vi "automated_scan_v1.2.vi"() -> ()   [LabVIEW 2018]
uses:
  Other_Libraries/MoCo Software/VI/global_m.vi
  <vilib>/Utility/file.llb/Write Delimited Spreadsheet (DBL).vi
  <vilib>/Utility/file.llb/Write Delimited Spreadsheet (string).vi
  Other_Libraries/Thorlabs_FW102C/Thorlabs_FW102C.lvlib
panel:
  out "Time per step":dbl
  out "Scan time(min)":dbl
  out "End scan":errorcluster
  out "FW Position":i32
  out "Filter Wheel":errorcluster
  out "Current Wavelength(nm)":dbl
  out "Take Image":errorcluster
  out "% complete":dbl
  out "Total Steps":dbl
  in  "Tab Control":T1(tab)
  in  "Mono port":refnum<visa-resource-name>="COM2"
  in  "Grating, gr/mm":u16(ring)=2 items=["2400", "1800", "1200", "600", "300", "150"]
  in  "Take Image":bool=TRUE
  in  "Two Cameras":bool=TRUE
  in  "Step Size":dbl=10.0
  in  "Stop Wavelength":dbl=600.0
  in  "Start Wavelength":dbl=500.0
  in  "Scan Directory":string="Peter_ferguson\\Tcal\\scans\\"
  in  "Scan Name":string="test_scan"
  in  "Scan Type":string(combo)="New Scan"
  in  "Camera\n Integration time":dbl=10.0
  in  "Spectrometer Integration time":dbl=0.001
  out "VISA out":refnum<visa-resource-name>
  out "Mono wav":dbl format="%.3f"
  out "Mono/Photodiode":errorcluster
  out "Step #":i32
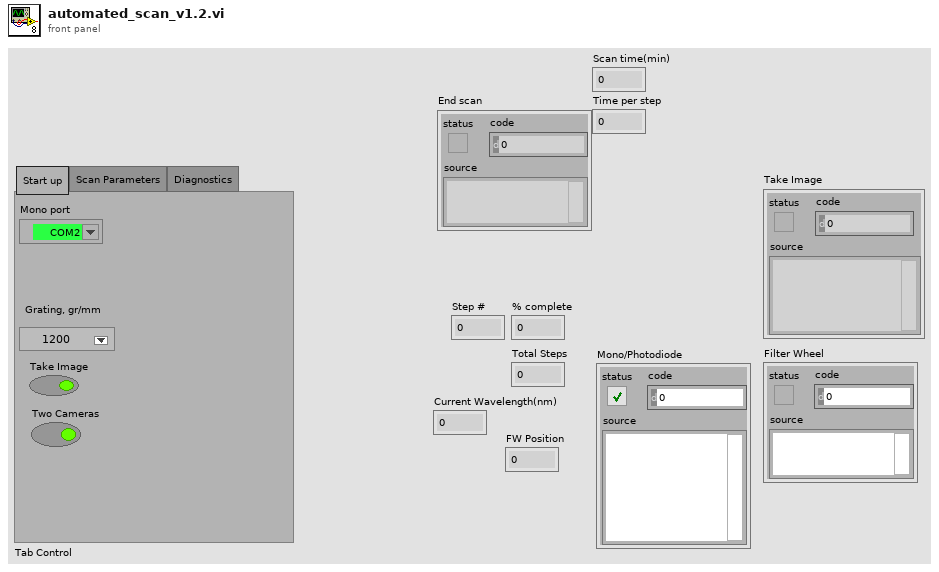
[diagram p1: front panel]
types:
  T1 = enum32{"Start up", "Scan Parameters", "Diagnostics"}
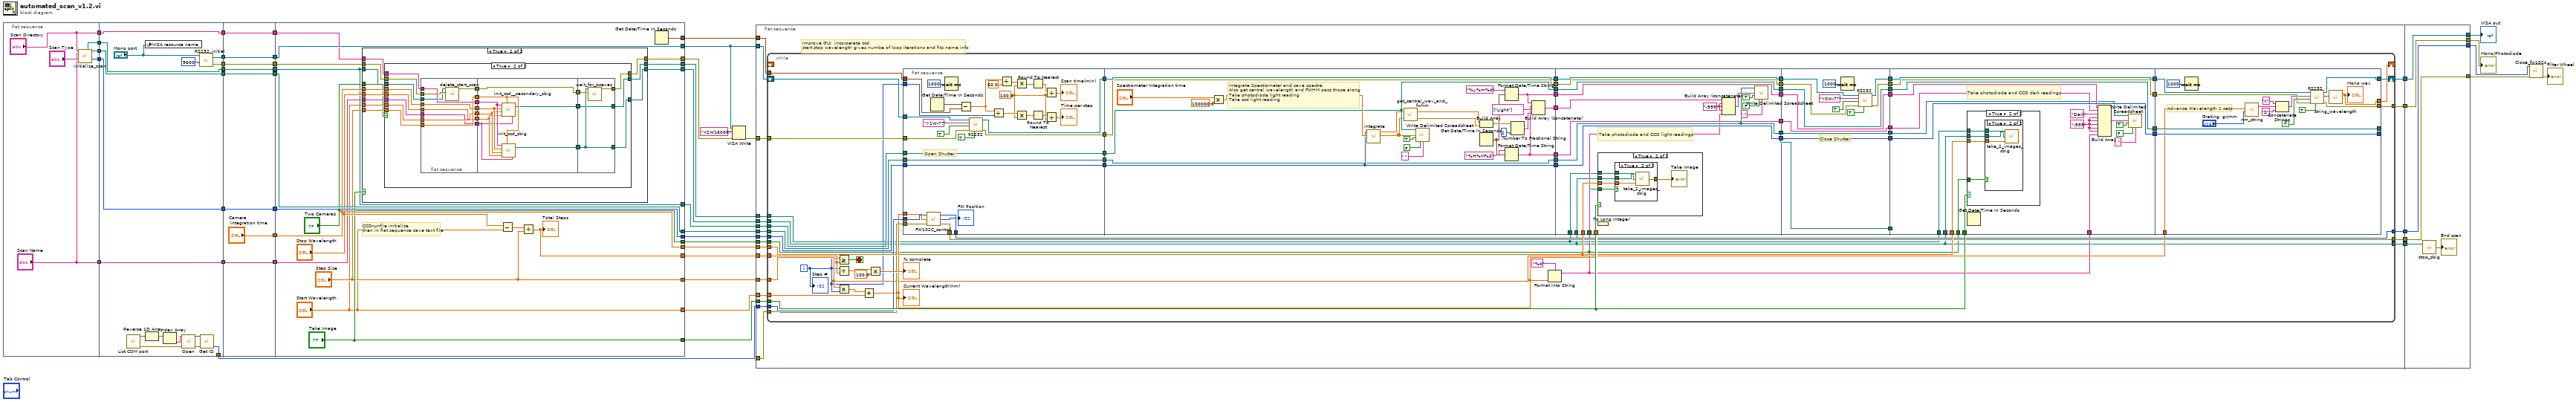
[diagram p0: block diagram]
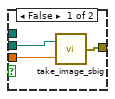
[diagram p3: hidden frame]
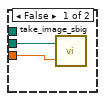
[diagram p5: hidden frame]
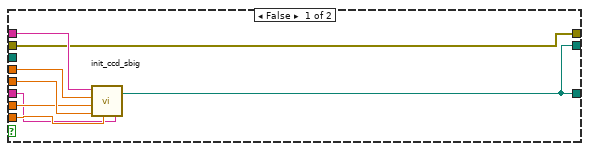
[diagram p7: hidden frame]
diagram:
  n1 = flat-sequence {
    tunnel: [w53] -> w39
    tunnel: [w52] -> w38
    tunnel: [w51] -> w37
    tunnel: ["Scan Directory"] -> w24
    tunnel: ["Scan Name"] -> w10
    tunnel: [w69] -> w36
    tunnel: [w68] -> w35
    tunnel: w39 -> [w67]
    tunnel: [w67] -> w34
    tunnel: w38 -> [w66]
    tunnel: [w66] -> w33
    tunnel: w37 -> [w65]
    tunnel: [w65] -> w32
    tunnel: w24 -> [w64]
    tunnel: [w64] -> w22
    tunnel: [w57] -> w17
    tunnel: [w56] -> w16
    tunnel: [w55] -> w11
    tunnel: w10 -> [w55]
    tunnel: w36 -> [w78]
    tunnel: [w78] -> w31
    tunnel: w35 -> [w72]
    tunnel: w34 -> [w77]
    tunnel: [w77] -> w30
    tunnel: w33 -> [w76]
    tunnel: [w76] -> w29
    tunnel: w32 -> [w75]
    tunnel: [w75] -> w28
    tunnel: ["Camera\n Integration time"] -> w27
    tunnel: [w72] -> w26
    tunnel: [w74] -> w23
    tunnel: w22 -> [w74]
    tunnel: [w73] -> w12
    tunnel: w11 -> [w73]
    tunnel: [w96] -> w41
    tunnel: w31 -> [w96]
    tunnel: [w88] -> w46
    tunnel: w30 -> [w88]
    tunnel: [w95] -> w45
    tunnel: w29 -> [w95]
    tunnel: [w94] -> w44
    tunnel: w28 -> [w94]
    tunnel: [w92] -> w43
    tunnel: w27 -> [w92]
    tunnel: [w97] -> w40
    tunnel: w26 -> [w84]
    tunnel: [w83] -> w25
    tunnel: w23 -> [w93]
    tunnel: [w90] -> w21
    tunnel: ["Take Image"] -> w20
    tunnel: ["Step Size"] -> w19
    tunnel: ["Start Wavelength"] -> w18
    tunnel: w12 -> [w85]
    tunnel: [w82] -> w4
    tunnel: ["Two Cameras"] -> w3
    tunnel: [w80] -> w1
    frame #0 {
      n2 = call "initialize_scan.vi"("Scan Directory"="Scan Directory", "Scan Name"="Scan Name", "Scan Type"="Scan Type") -> ("Path Spec"=w53:path, "Path Scan"=w51:path, "Wrapper Out"=w52:u64)  [unwired: 8 in, 2 out]
    }
    frame #1 {
      n3 = call "List COM port.vi"() -> ("error out"=w58:errorcluster, "COM Ports"=w61:string[])  [unwired: 10 in]
      n4 = global write "global_m.vi" "VISA resource name"("Mono port") -> ()
      n5 = Reverse 1D Array(array=w61) -> (reversed array=w60:string[])
      n6 = Index Array(array=w60) -> (element=w59:string)  [unwired: 1 in]
      n7 = call "Open.vi"("error in (no error)"=w58, "Serial Port"=w59) -> ("error out"=w62:errorcluster, "FW102C out"=w63:i32)  [unwired: 7 in, 1 out]
      n8 = call "RS232_initial.vi"("baud rate"=u32 9600, "VISA resource name"="Mono port") -> ("error out"=w68:errorcluster, "VISA name out"=w69:refnum<visa-resource-name>)  [unwired: 2 in]
      n9 = call "Get ID.vi"("error in (no error)"=w62, "FW102C in"=w63) -> ("error out"=w56:errorcluster, "FW102C out"=w57:i32)  [unwired: 7 in, 1 out]
    }
    frame #2 {
    }
    frame #3 {
      # "CCDrunfile initialize\nthen in flat sequence save text file"
      n10 = case shown="True" "Take Image" {
        tunnel: w93 -> [_ w112]
        tunnel: w92 -> [_ w111]
        tunnel: "Step Size" -> [_ w110]
        tunnel: "Stop Wavelength" -> [_ w109]
        tunnel: [w99 w108] -> w90
        tunnel: "Start Wavelength" -> [_ w107]
        tunnel: w88 -> [w99 w102]
        tunnel: "Two Cameras" -> [_ w106]
        tunnel: w85 -> [_ w105]
        tunnel: w84 -> [w100 w104]
        tunnel: [w100 w103] -> w83
        tunnel: [w99 w101] -> w82
        frame False {
        }
        frame True {
          n11 = case shown="True" w106 {
            tunnel: w112 -> [w120 w139]
            tunnel: w111 -> [w119 w138]
            tunnel: w110 -> [w118 w140]
            tunnel: w109 -> [w117 w136]
            tunnel: [w113 w141] -> w108
            tunnel: w107 -> [w116 w137]
            tunnel: w105 -> [w115 w135]
            tunnel: w104 -> [w114 w126]
            tunnel: [w114 w133] -> w103
            tunnel: w102 -> [_ w123]
            tunnel: [w113 w121] -> w101
            frame False {
              n12 = call "init_ccd_sbig.vi"("Scan Directory"=w120, "Exposure Time"=w119, "Min nm"=w116, "Max nm"=w117, "Step size"=w118, "Scan_prefix"=w115) -> ("Working Directory"=w113:path)
            }
            frame True {
              n13 = flat-sequence {
                tunnel: w135 -> [w145]
                tunnel: w136 -> [w146]
                tunnel: w137 -> [w147]
                tunnel: w138 -> [w148]
                tunnel: w139 -> [w149]
                tunnel: w140 -> [w150]
                tunnel: [w150] -> w132
                tunnel: [w149] -> w131
                tunnel: [w148] -> w130
                tunnel: [w147] -> w129
                tunnel: [w146] -> w128
                tunnel: [w145] -> w127
                tunnel: w126 -> [w144]
                tunnel: [w143] -> w124
                tunnel: w123 -> [w142]
                tunnel: [w153] -> w134
                tunnel: w132 -> [w159]
                tunnel: w131 -> [w158]
                tunnel: w130 -> [w157]
                tunnel: w129 -> [w156]
                tunnel: w128 -> [w155]
                tunnel: w127 -> [w154]
                tunnel: [w152] -> w125
                tunnel: w124 -> [w152]
                tunnel: [w151] -> w122
                tunnel: [w162] -> w141
                tunnel: w134 -> [w162]
                tunnel: [w163] -> w133
                tunnel: w125 -> [w161]
                tunnel: w122 -> [w160]
                tunnel: [w160] -> w121
                frame #0 {
                  n14 = call "delete_start_scan.vi"("error out"=w144, "base path"=w142) -> ("error out 2"=w143:errorcluster)  [unwired: 9 in]
                }
                frame #1 {
                  n15 = call "init_ccd__secondary_sbig.vi"("Scan Directory"=w158, "Exposure Time"=w157, "Min nm"=w156, "Max nm"=w155, "Step size"=w159, "Scan_prefix"=w154) -> ("Working Directory"=w151:path)
                  n16 = call "init_ccd_sbig.vi"("Scan Directory"=w158, "Exposure Time"=w157, "Min nm"=w156, "Max nm"=w155, "Step size"=w159, "Scan_prefix"=w154) -> ("Working Directory"=w153:path)
                }
                frame #2 {
                  n17 = call "wait_for_psexec.vi"("error out"=w161, "base path"=w162) -> ("error out 2"=w163:errorcluster)  [unwired: 9 in]
                }
              }
            }
          }
        }
      }
      n18 = Subtract(x="Stop Wavelength", y="Start Wavelength") -> (x-y=w98:dbl)
      n19 = Divide(x=w98, y="Step Size") -> (x/y=w97:dbl)
      "Total Steps" <- w97
      n20 = Get Date/Time In Seconds() -> (seconds since 1Jan1904=w80:timestamp)
    }
  }
  n21 = VISA Write(VISA resource name=w41, write buffer="X2W1600R", error in (no error)=w25) -> (error out=w47:errorcluster)  [unwired: 2 out]
  n22 = flat-sequence {
    tunnel: w47 -> [w184]
    tunnel: w46 -> [w183]
    tunnel: w45 -> [w182]
    tunnel: w44 -> [w181]
    tunnel: w43 -> [w180]
    tunnel: w41 -> [w177]
    tunnel: w40 -> [w176]
    tunnel: w21 -> [w175]
    tunnel: w20 -> [w174]
    tunnel: w19 -> [w173]
    tunnel: w18 -> [w172]
    tunnel: w17 -> [w171]
    tunnel: w16 -> [w170]
    tunnel: [w179] -> w9
    tunnel: [w178] -> w8
    tunnel: [w169] -> w7
    tunnel: [w168] -> w6
    tunnel: [w167] -> w5
    tunnel: w4 -> [w166]
    tunnel: w3 -> [w165]
    tunnel: w1 -> [w164]
    tunnel: [w395] -> w13
    tunnel: [w396] -> w14
    tunnel: [w397] -> w42
    tunnel: [w398] -> w2
    tunnel: w9 -> [w398]
    tunnel: w8 -> [w397]
    tunnel: w7 -> [w396]
    tunnel: w6 -> [w395]
    tunnel: w5 -> [w394]
    frame #0 {
      # "Improve GUI, incorperate ccd,\nstart stop wavelength gives numbe of loop iterations and fits name info"
      n23 = while {
        tunnel: w184 -> [w246]
        tunnel: [w245] -> w179
        tunnel: w183 -> [w244]
        tunnel: w182 -> [w243]
        shift-right: [w206] -> _
        shift-left: _ -> [_]
        tunnel: w181 -> [w230]
        tunnel: w180 -> [w198]
        shift-right: [w208] -> w178
        shift-left: w177 -> [w207]
        tunnel: w176 -> [w205]
        tunnel: w175 -> [w189]
        tunnel: w174 -> [w201]
        tunnel: w173 -> [w190]
        tunnel: w172 -> [w200]
        tunnel: w171 -> [w196]
        tunnel: w170 -> [w195]
        tunnel: [w193] -> w168
        tunnel: [w192] -> w169
        tunnel: [w189] -> w167
        tunnel: w166 -> [w188]
        tunnel: w165 -> [w187]
        tunnel: w164 -> [w186]
        i -> [w185]
        stop <- w216 stop-if-true
        n24 = Greater Or Equal?(x=w185, y=w205) -> (x >= y?=w216:bool)
        n25 = Divide(x=w185, y=w205) -> (x/y=w204:dbl)
        n26 = Multiply(x=w190, y=w185) -> (x*y=w199:dbl)
        n27 = Add(x=w199, y=w200) -> (x+y=w194:dbl)
        "Current Wavelength(nm)" <- w194
        n28 = Multiply(x=w204, y=100.0) -> (x*y=→"% complete":dbl)
        n29 = flat-sequence {
          tunnel: w246 -> [w276]
          tunnel: [w275] -> w242
          tunnel: [w274] -> w241
          tunnel: [w270] -> w240
          tunnel: w244 -> [w270]
          tunnel: w243 -> [w269]
          tunnel: [w269] -> w239
          tunnel: w230 -> [w268]
          tunnel: [w268] -> w229
          tunnel: w207 -> [w267]
          tunnel: w196 -> [w266]
          tunnel: w195 -> [w265]
          tunnel: w194 -> [w264]
          tunnel: [w263] -> w193
          tunnel: [w262] -> w192
          tunnel: w186 -> [w259]
          tunnel: w185 -> [w258]
          tunnel: w242 -> [w302]
          tunnel: [w302] -> w228
          tunnel: w241 -> [w301]
          tunnel: [w301] -> w227
          tunnel: w240 -> [w293]
          tunnel: [w293] -> w226
          tunnel: w239 -> [w294]
          tunnel: [w294] -> w224
          tunnel: w229 -> [w282]
          tunnel: [w282] -> w222
          tunnel: [w281] -> w221
          tunnel: [w279] -> w215
          tunnel: [w278] -> w210
          tunnel: w228 -> [w320]
          tunnel: w227 -> [w314]
          tunnel: w226 -> [w322]
          tunnel: [w322] -> w225
          tunnel: w224 -> [w321]
          tunnel: [w321] -> w223
          tunnel: w222 -> [w313]
          tunnel: w221 -> [w316]
          tunnel: [w320] -> w220
          tunnel: w198 -> [w309]
          tunnel: [w314] -> w219
          tunnel: [w313] -> w218
          tunnel: w215 -> [w312]
          tunnel: [w312] -> w214
          tunnel: [w311] -> w211
          tunnel: w210 -> [w311]
          tunnel: w189 -> [w310]
          tunnel: w201 -> [w308]
          tunnel: w191 -> [w306]
          tunnel: w194 -> [w307]
          tunnel: w188 -> [w305]
          tunnel: w187 -> [w304]
          tunnel: [w346] -> w238
          tunnel: [w345] -> w236
          tunnel: w225 -> [w341]
          tunnel: [w341] -> w234
          tunnel: [w340] -> w232
          tunnel: w223 -> [w340]
          tunnel: w220 -> [w339]
          tunnel: w219 -> [w338]
          tunnel: w218 -> [w335]
          tunnel: [w335] -> w217
          tunnel: w214 -> [w337]
          tunnel: [w337] -> w213
          tunnel: [w336] -> w212
          tunnel: w211 -> [w336]
          tunnel: [w335] -> w209
          tunnel: w238 -> [w366]
          tunnel: [w366] -> w237
          tunnel: w236 -> [w365]
          tunnel: [w365] -> w235
          tunnel: w234 -> [w364]
          tunnel: [w364] -> w233
          tunnel: w232 -> [w363]
          tunnel: [w363] -> w231
          tunnel: w217 -> [_]
          tunnel: w198 -> [w354]
          tunnel: w213 -> [w357]
          tunnel: w212 -> [w356]
          tunnel: w209 -> [w355]
          tunnel: w189 -> [w353]
          tunnel: w201 -> [w352]
          tunnel: w191 -> [w351]
          tunnel: w188 -> [w350]
          tunnel: w187 -> [w349]
          tunnel: w237 -> [w389]
          tunnel: w235 -> [w390]
          tunnel: w233 -> [w379]
          tunnel: w231 -> [w381]
          tunnel: [w388] -> w208
          tunnel: [w387] -> w245
          tunnel: [w381] -> _
          tunnel: [w379] -> _
          tunnel: [w378] -> w206
          tunnel: w190 -> [w377]
          frame #0 {
            w249 = 100.0 ("y")
            # "Open Shutter"
            n30 = call "FW102C_control.vi"("error in (no error)"=w265, "Current Wavelength"=w264, "FW102C in"=w266) -> ("error out"=w262:errorcluster, "Position"=→"FW Position":i32, "FW102C out"=w263:i32)
            n31 = Get Date/Time In Seconds() -> (seconds since 1Jan1904=w260:timestamp)
            n32 = Wait (ms)(milliseconds to wait=u32 1000) -> ()  [unwired: 1 out]
            n33 = Subtract(x=w260, y=w259) -> (x-y=w257:dbl)
            n34 = call "RS232.vi"("read"=TRUE, "error in"=w276, "write"=TRUE, "string to write"="Y1W-7?" ("string"), "VISA  name in"=w267) -> ("error out"=w274:errorcluster, "VISA out"=w275:refnum<visa-resource-name>)  [unwired: 1 in, 2 out]
            n35 = Divide(x=w257, y=w258) -> (x/y=w255:dbl)
            n36 = Divide(x=w257, y=60.0) -> (x/y=w251:dbl)
            n37 = Multiply(x=w251, y=w249) -> (x*y=w250:dbl)
            n38 = Multiply(x=w255, y=w249) -> (x*y=w254:dbl)
            n39 = Round To Nearest(number=w250) -> (nearest integer value=w248:dbl)
            n40 = Round To Nearest(number=w254) -> (nearest integer value=w253:dbl)
            n41 = Divide(x=w248, y=w249) -> (x/y=→"Scan time(min)":dbl)
            n42 = Divide(x=w253, y=w249) -> (x/y=→"Time per step":dbl)
          }
          frame #1 {
            # "Integrate Spectrometer and save spectra, \nAlso get central wavelength and FWHM pass those along\nTake photodiode light reading \nTake ccd light reading"
            n43 = Multiply(x="Spectrometer Integration time", y=100000.0) -> (x*y=w298:dbl)
            n44 = call "integrate.vi"("Numeric"=w298, "Wrapper Out"=w294) -> ("Spectrum Values"=w291:dbl[], "WL Values"=w292:dbl[])  [unwired: 7 in, 1 out]
            n45 = call "get_central_wav_and_fwhm.vi"("Signal"=w291, "Wavelenghs"=w292) -> ("FWHM"=w287:dbl, "Central"=w280:dbl)
            n46 = call-poly <vilib>:"Write Delimited Spreadsheet.vi"("file path (dialog if empty)"=w293, "1D data"=w291, "append to file? (new file:F)"=TRUE, "transpose? (no:F)"=FALSE, "delimiter (\\t)"="," ("delimiter (\\t)")) -> ()  [unwired: 9 in, 2 out]
            n47 = Build Array(w280, w287) -> (w286:dbl[])
            n48 = Get Date/Time In Seconds() -> (seconds since 1Jan1904=w289:timestamp)
            n49 = Format Date/Time String(time format string (%c)="%y%m%d", seconds (now)=w289) -> (date/time string=w279:string)  [unwired: 1 in]
            n50 = Format Date/Time String(time format string (%c)="%H%M%S", seconds (now)=w289) -> (date/time string=w278:string)  [unwired: 1 in]
            n51 = Number To Fractional String(number=w286, precision (6)=i16 2) -> (F-format string=w283:string[])  [unwired: 2 in]
            n52 = Build Array (concatenate)(w279, w278, string[] ["Light"] ("array"), w283) -> (w281:string[])
          }
          frame #2 {
            w303 = "-999" ("element")
            # "Take photodiode and CCD light readings"
            n53 = To Long Integer(number=w307) -> ()  [unwired: 1 out]
            n54 = case shown="True" w308 {
              tunnel: w310 -> [_ w327]
              tunnel: w309 -> [_ w326]
              tunnel: w305 -> [_ w325]
              tunnel: w304 -> [_ w323]
              frame False {
              }
              frame True {
                n55 = case shown="True" w323 {
                  tunnel: w327 -> [w330 w333]
                  tunnel: w326 -> [w329 w334]
                  tunnel: w325 -> [_ w332]
                  tunnel: [w328 w331] -> w324
                  frame False {
                    n56 = call "take_image_sbig.vi"("Exptime"=w329, "path"=w330) -> ("error out"=w328:errorcluster)
                  }
                  frame True {
                    n57 = call "take_2_images_sbig.vi"("Exptime"=w334, "secondary path"=w332, "primary_path"=w333) -> ("error out"=w331:errorcluster)
                  }
                }
                "Take Image" <- w324
              }
            }
            n58 = Build Array (concatenate)(w316, w303, w303, w303, w306) -> (w315:string[])
            n59 = call-poly <vilib>:"Write Delimited Spreadsheet.vi"("file path (dialog if empty)"=w313, "1D data"=w315, "append to file? (new file:F)"=TRUE, "transpose? (no:F)"=FALSE, "delimiter (\\t)"="," ("delimiter (\\t)")) -> ()  [unwired: 9 in, 2 out]
          }
          frame #3 {
            # "Close Shutter"
            n60 = Wait (ms)(milliseconds to wait=u32 1000) -> ()  [unwired: 1 out]
            n61 = call "RS232.vi"("read"=TRUE, "error in"=w338, "write"=TRUE, "string to write"="Y0W-7?" ("string"), "VISA  name in"=w339) -> ("error out"=w345:errorcluster, "VISA out"=w346:refnum<visa-resource-name>)  [unwired: 1 in, 2 out]
          }
          frame #4 {
            w348 = "-999" ("element")
            # "Take photodiode and CCD dark readings"
            n62 = case shown="True" w352 {
              tunnel: w354 -> [_ w370]
              tunnel: w353 -> [_ w369]
              tunnel: w350 -> [_ w368]
              tunnel: w349 -> [_ w367]
              frame False {
              }
              frame True {
                n63 = case shown="True" w367 {
                  tunnel: w370 -> [w372 w374]
                  tunnel: w369 -> [w371 w375]
                  tunnel: w368 -> [_ w373]
                  frame False {
                    n64 = call "take_image_sbig.vi"("Exptime"=w372, "path"=w371) -> ()  [unwired: 1 out]
                  }
                  frame True {
                    n65 = call "take_2_images_sbig.vi"("Exptime"=w374, "secondary path"=w373, "primary_path"=w375) -> ()  [unwired: 1 out]
                  }
                }
              }
            }
            n66 = Get Date/Time In Seconds() -> ()  [unwired: 1 out]
            n67 = Build Array(w357, w356, "Dark" ("date/time string"), w348, w348, w348, w348, w348, w351) -> (w358:string[])
            n68 = call-poly <vilib>:"Write Delimited Spreadsheet.vi"("file path (dialog if empty)"=w355, "1D data"=w358, "append to file? (new file:F)"=TRUE, "transpose? (no:F)"=FALSE, "delimiter (\\t)"="," ("delimiter (\\t)")) -> ()  [unwired: 9 in, 2 out]
          }
          frame #5 {
            # "Advance Wavelength 1 setp"
            n69 = Wait (ms)(milliseconds to wait=u32 1000) -> ()  [unwired: 1 out]
            n70 = call "nm_string.vi"("Grating, gr/mm"="Grating, gr/mm", "Wavelength, nm"=w377) -> ("nm_String"=w386:string)  [unwired: 2 in, 1 out]
            n71 = Concatenate Strings("X" ("string"), w386, "S" ("string")) -> (w383:string)
            n72 = call "RS232.vi"("read"=TRUE, "error in"=w390, "write"=TRUE, "string to write"=w383, "VISA  name in"=w389) -> ("error out"=w387:errorcluster, "read string"=w380:string, "VISA out"=w388:refnum<visa-resource-name>)  [unwired: 1 in, 1 out]
            n73 = call "string_wavelength.vi"("Position String"=w380) -> ("Present Wavelength"=w378:dbl)  [unwired: 3 in, 1 out]
            "Mono wav" <- w378
          }
        }
        n74 = Format Into String(format string="%d", w194) -> (resulting string=w191:string)  [unwired: 2 in, 1 out]
        "Step #" <- w185
      }
    }
    frame #1 {
      n75 = call "stop_sbig.vi"("path"=w394) -> ("error out"=→"End scan":errorcluster)  [unwired: 1 in]
    }
  }
  n76 = call "Close_fw102c.vi"("error in (no error)"=w14, "FW102C in"=w13) -> ("error out"=→"Filter Wheel":errorcluster)  [unwired: 9 in]
  "Mono/Photodiode" <- w2
  "VISA out" <- w42
